vi "util.ntr.dose-path.vi"(10 "ntrGraphPeriod":T2 {"Time range"."Start" format="%<%H:%M %d/%m/%y>T"; "Time range"."End" format="%<%H:%M %d/%m/%y>T"}, 11 "Dosepump":string) -> (0 "error out":errorcluster, 2 "Graph":cluster{"X":dbl[], "Y":dbl[]}(graph), 3 "Filenames":string[](array[string]))   [LabVIEW 2024]
uses:
  controls/UiScheduleTimestamp.ctl
  controls/typePathSelector.ctl
  <vilib>/Utility/error.llb/Clear Errors.vi
  <vilib>/Utility/libraryn.llb/Create Directory Recursive.vi
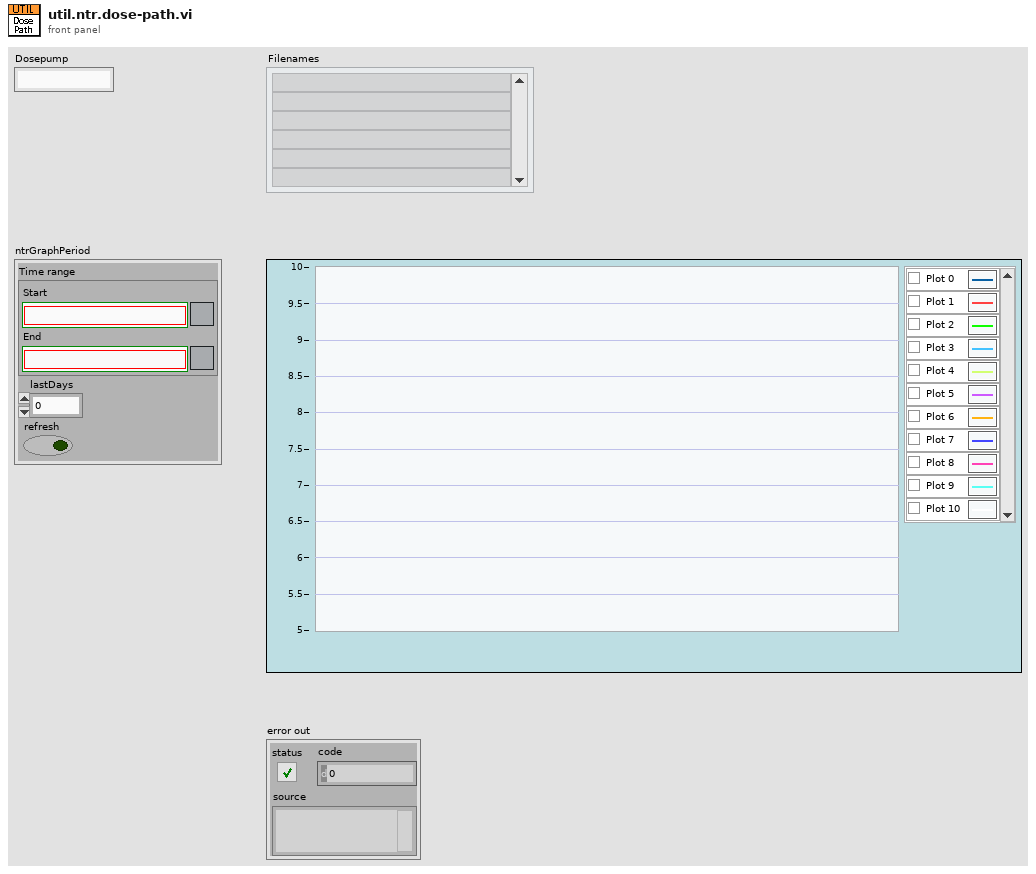
[diagram p1: front panel]
types:
  T1 = typedef "UiScheduleTimestamp.ctl" = timestamp
  T2 = cluster{"Time range":cluster{"Start":T1, "End":T1}, "lastDays":dbl, "refresh":bool}
  T3 = typedef "typePathSelector.ctl" = enum16{"DIR_PROCS", "DIR_CONFIG", "DIR_TEMPLATE", "DIR_IO_FILE", "DIR_RECORD", "DIR_LOG", "DIR_RUNTIME", "DIR_PRESET", "DIR_INI"}
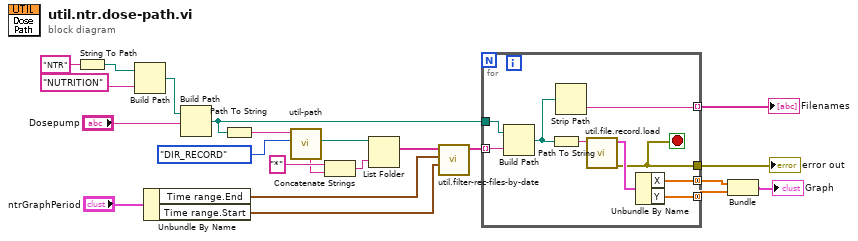
[diagram p0: block diagram]
diagram:
  n1 = String To Path(string="NTR" ("append path (ie. folder\\filename.*)")) -> (path=w3:path)
  n2 = Build Path(base path=w3, name or relative path="NUTRITION" ("append path (ie. folder\\filename.*)")) -> (appended path=w1:path)
  n3 = Unbundle By Name("ntrGraphPeriod") -> ("Time range.End"=w20:T1, "Time range.Start"=w21:T1)
  n4 = Build Path(base path=w1, name or relative path="Dosepump") -> (appended path=w5:path)
  n5 = Path To String(path=w5) -> (string=w14:string)
  n6 = call "util-path.vi"("Selected Folder (PROCS)"=typePathSelector."DIR_RECORD" ("Selected Folder (PROCEDURE_DIR)"), "append path (ie. folder\\filename.*)"=w14) -> ("SelectedPath"=w18:path, ".extension (.prc)"=w15:string)  [unwired: 5 in, 3 out]
  n7 = Concatenate Strings("*" ("string"), w15) -> (w16:string)
  n8 = List Folder(path=w18, pattern=w16) -> (filenames=w19:string[])  [unwired: 2 in, 3 out]
  n9 = call "util.filter-rec-files-by-date.vi"("Date Start"=w21, "Date End"=w20, "filenames"=w19) -> ("Array"=w6:string[])  [unwired: 7 in, 1 out]
  n10 = for {
    tunnel: w6 -> [w31] mode=indexing
    tunnel: w5 -> [w30]
    tunnel: [w23] -> w10 mode=indexing
    tunnel: [w27] -> w9 mode=concatenating
    tunnel: [w26] -> w8 mode=concatenating
    tunnel: [w25] -> w4
    stop <- w25 stop-if-true
    n11 = Build Path(base path=w30, name or relative path=w31) -> (appended path=w24:path)
    n12 = Path To String(path=w24) -> (string=w29:string)
    n13 = Strip Path(path=w24) -> (name=w23:string)  [unwired: 1 out]
    n14 = call "util.file.record.load.vi"("filename.*"=w29) -> ("error out"=w25:errorcluster, "Multiple Plots (X Array and Y Array) 2"=w28:cluster{"X":dbl[], "Y":dbl[]})  [unwired: 8 in, 1 out]
    n15 = Unbundle By Name(w28) -> ("X"=w27:dbl[], "Y"=w26:dbl[])
  }
  "Filenames" <- w10
  "error out" <- w4
  n16 = Bundle("X"=w9, "Y"=w8) -> (→"Graph":cluster{"X":dbl[], "Y":dbl[]})  [unwired: 1 in]
